vi "采集.vi"() -> ()   [LabVIEW 2018]
uses:
  <vilib>/Instr/_visa.llb/VISA Configure Serial Port (Instr).vi
panel:
  out "通讯中":bool[](array[boolean])
  out "采集到的波形":dbl[](graph)
  in  "停止":bool
  in  "采集":bool
  # "地学虚拟仪器采集模块"
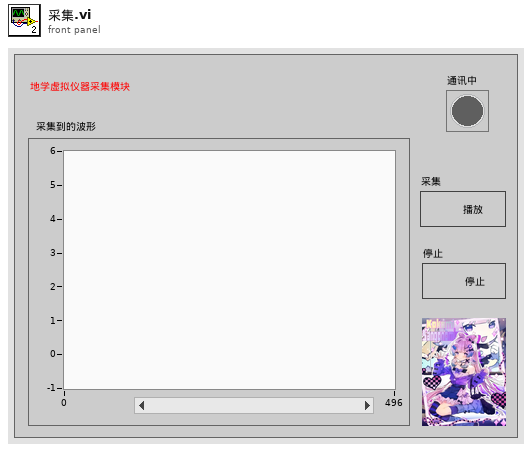
[diagram p1: front panel]
types:
  T1 = enum16{"open", "replace", "create", "open or create", "replace or create", "replace or create with confirmation"}
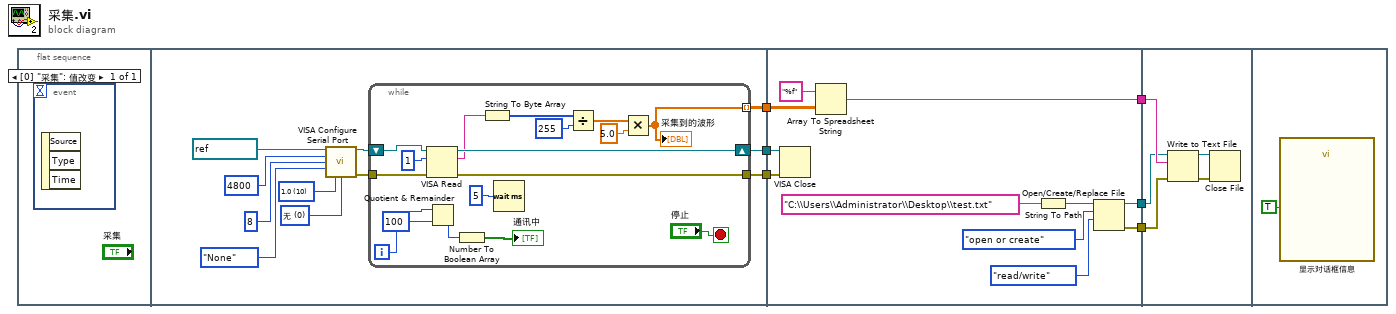
[diagram p0: block diagram]
diagram:
  n1 = flat-sequence {
    tunnel: [w8] -> w6
    tunnel: [w9] -> w5
    tunnel: [w7] -> w4
    tunnel: w6 -> [w45]
    tunnel: w5 -> [w44]
    tunnel: w4 -> [w43]
    tunnel: [w37] -> w3
    tunnel: [w36] -> w2
    tunnel: [w35] -> w1
    tunnel: w3 -> [w50]
    tunnel: w2 -> [w49]
    tunnel: w1 -> [w48]
    frame #0 {
      n2 = event shown="[0] \"采集\": 值改变" {
        selector: _ -> [_]
        dyn-events: _ -> [_]
        timeout: _ -> [_]
        event "采集": Value Change {
          n3 = event-data() -> ()  [unwired: 1 in, 3 out]
        }
      }
    }
    frame #1 {
      w10 = u16 0 items=["无", "XON/XOFF", "RTS/CTS", "XON/XOFF & RTS/CTS", "DTR/DSR", "XON/XOFF & DTR/DSR"] ("flow control (0:none)")
      w11 = u16 10 items=["1.0"=10, "1.5"=15, "2.0"=20] ("stop bits (10: 1 bit)")
      n4 = call-poly "VISA Configure Serial Port"("VISA resource name"=refnum<visa-resource-name> "COM1", "baud rate (9600)"=u32 4800, "data bits (8)"=u16 8, "parity (0:none)"=enum16{"None", "Odd", "Even", "Mark", "Space"}."None", "stop bits (10: 1 bit)"=w11, "flow control (0:none)"=w10) -> ("VISA resource name out"=w17:refnum<visa-resource-name>, "error out"=w16:errorcluster)  [unwired: 8 in]
      n5 = while {
        shift-right: [w33] -> w9
        shift-left: w17 -> [w31]
        tunnel: w16 -> [w30]
        tunnel: [w32] -> w8
        tunnel: [w22] -> w7 mode=indexing
        i -> [w20]
        stop <- "停止" stop-if-true
        n6 = VISA Read(VISA resource name=w31, byte count=u32 1 ("字节总数"), error in (no error)=w30) -> (VISA resource name out=w33:refnum<visa-resource-name>, read buffer=w28:string, error out=w32:errorcluster)  [unwired: 1 out]
        n7 = Quotient & Remainder(x=w20, y=100) -> (floor(x/y)=w18:i32)  [unwired: 1 out]
        n8 = Number To Boolean Array(number=w18) -> (Boolean array=→"通讯中":bool[])
        n9 = String To Byte Array(string=w28) -> (unsigned byte array=w27:u8[])
        n10 = Wait (ms)(milliseconds to wait=u32 5 ("等待时间（毫秒）")) -> ()  [unwired: 1 out]
        n11 = Divide(x=w27, y=255) -> (x/y=w25:dbl[])
        n12 = Multiply(x=w25, y=5.0) -> (x*y=w22:dbl[])
        "采集到的波形" <- w22
      }
    }
    frame #2 {
      n13 = VISA Close(VISA resource name=w44, error in (no error)=w45) -> ()  [unwired: 1 out]
      n14 = Array To Spreadsheet String(array=w43, 3:"%f" ("格式字符串")) -> (spreadsheet string=w37:string)  [unwired: 1 in]
      n15 = String To Path(string="C:\\Users\\Administrator\\Desktop\\test.txt") -> (path=w40:path)
      n16 = Open/Create/Replace File(file path (use dialog)=w40, operation (0:open)=T1."open or create" ("操作(0:open)"), access (0:read/write)=enum16{"read/write", "read-only", "write-only"}."read/write" ("权限(0:read/write)")) -> (refnum out=w36:refnum<file>, error out=w35:errorcluster)  [unwired: 3 in, 1 out]
    }
    frame #3 {
      n17 = Write to Text File(file (use dialog)=w49, text=w50, error in=w48) -> (refnum out=w46:refnum<file>, error out=w47:errorcluster)  [unwired: 1 in, 1 out]
      n18 = Close File(refnum=w46, error in=w47) -> ()  [unwired: 2 out]
    }
    frame #4 {
      n19 = call "显示对话框信息"("Enable"=TRUE) -> ()  [unwired: 9 in, 2 out]
    }
  }
